vi "Stop&Close(Utility).vi"(8 "error in (no error)":errorcluster) -> (0 "error out":errorcluster)   [LabVIEW 2013, in "OPCUA(UtilityMode).lvlib"]
uses:
  OPCUA(UtilityMode).lvlib
  op(utility).ctl
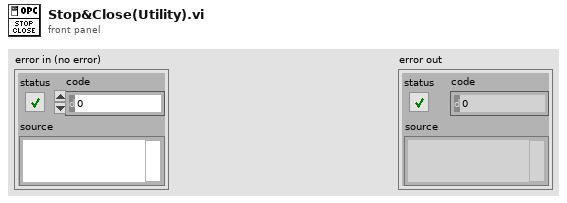
[diagram p1: front panel]
types:
  T1 = typedef "OPCUA(UtilityMode).lvlib/op(utility).ctl" = enum16{"Create Server", "Start Server", "Get Server Refnum", "Stop Server", "Close Server"}
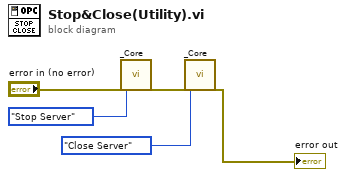
[diagram p0: block diagram]
diagram:
  n1 = call "_Core.vi"("error in (no error)"="error in (no error)", "Op"=op(utility)."Stop Server") -> ("error out"=w2:errorcluster)  [unwired: 21 in, 4 out]
  n2 = call "_Core.vi"("error in (no error)"=w2, "Op"=op(utility)."Close Server") -> ("error out"=→"error out":errorcluster)  [unwired: 21 in, 4 out]
